vi "ConfigureInputGpio.vi"(8 "error in (no error)":errorcluster, 10 "Pin":i32, 11 "connection ID":refnum<k5>) -> (0 "error out":errorcluster, 3 "connection ID out":refnum<k5>)   [LabVIEW 2023, in "Numato.lvlib"]
uses:
  Numato.lvlib
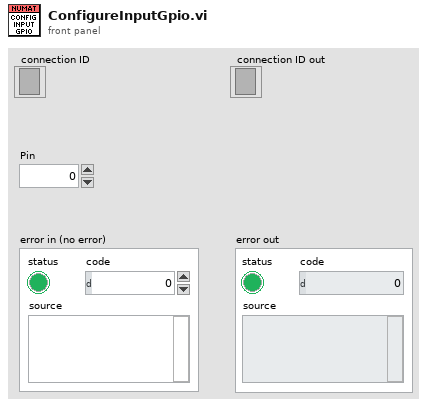
[diagram p1: front panel]
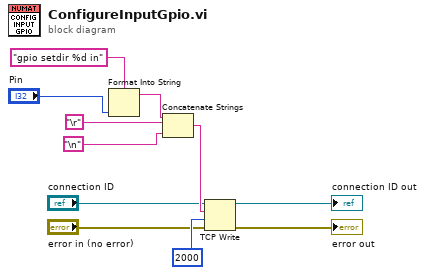
[diagram p0: block diagram]
diagram:
  n1 = Format Into String(format string="gpio setdir %d in" ("data in"), "Pin") -> (resulting string=w1:string)  [unwired: 2 in, 1 out]
  n2 = Concatenate Strings(w1, "\r", "\n") -> (w10:string)
  n3 = TCP Write(connection ID="connection ID", data in=w10, error in (no error)="error in (no error)", 9:2000 ("timeout ms (25000)")) -> (connection ID out=→"connection ID out":refnum<k5>, error out=→"error out":errorcluster)  [unwired: 1 out]
